vi "Initialize Queue Log.vi"(7 "context":string, 8 "error in (no error)":errorcluster, 9 "queue in (default: new queue)":refnum<queue>, 10 "level":T1 items=["OFF"=0, "FATAL"=100, "ERROR"=200, "WARN"=300, "INFO"=400, "DEBUG"=500, "TRACE"=600, "ALL"=65535]) -> (0 "error out":errorcluster, 1 "queue out":refnum<queue>, 3 "Queue Log Provider out":refnum<class "Queue Log Provider.lvclass">)   [LabVIEW 2019, in "Queue Log Provider.lvclass"]
uses:
  Queue Log Provider.lvclass
  Log Service/public/level.ctl
  Log Service/Log Service.lvclass
  impl/log_message.ctl
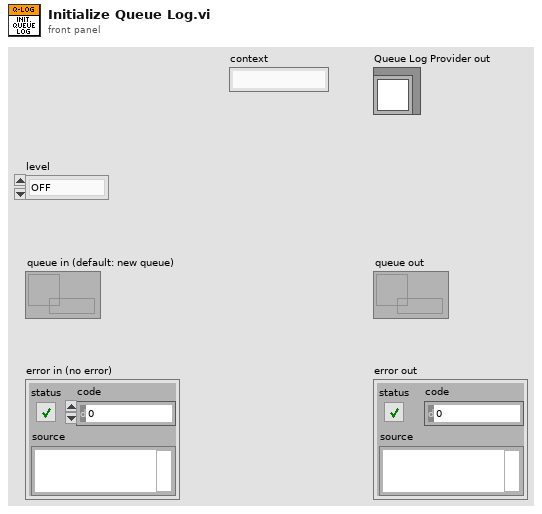
[diagram p1: front panel]
types:
  T1 = typedef "Utility API.lvlib/Log Service.lvclass/level.ctl" = u16
  T2 = typedef "Queue Log Provider.lvclass/log_message.ctl" = cluster{"Time Stamp":timestamp, "level":T1, "context":string, "message":string}
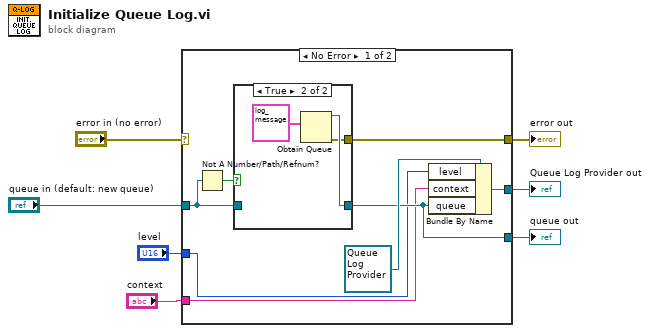
[diagram p0: block diagram]
diagram:
  n1 = case shown="No Error" "error in (no error)" {
    selector: "error in (no error)" -> [_ w21]
    tunnel: [w14 _] -> w7
    tunnel: [w13 w21] -> w6
    tunnel: [w12 w20] -> w5
    tunnel: "queue in (default: new queue)" -> [w11 w20]
    tunnel: "level" -> [w10 _]
    tunnel: "context" -> [w9 _]
    frame No Error {
      n2 = Not A Number/Path/Refnum?(number/path/refnum=w11) -> (NaN/Path/Refnum?=w8:bool)
      n3 = case shown="True" w8 {
        tunnel: [w16 w18] -> w12
        tunnel: w11 -> [w16 _]
        tunnel: [_ w17] -> w13
        frame False {
        }
        frame True {
          n4 = Obtain Queue(element data type=T2 {"Time Stamp"=timestamp(0 s since 1904-01-01), "level"=0, "context"="", "message"=""} ("message")) -> (queue out=w18:refnum<queue>, error out=w17:errorcluster)  [unwired: 4 in, 1 out]
        }
      }
      n5 = Bundle By Name(cluster=refnum<class "Queue Log Provider.lvclass"> refnum ("Queue Log Provider in"), "level"=w10, "context"=w9, "queue"=w12) -> (w14:refnum<class "Queue Log Provider.lvclass">)
    }
    frame Error {
    }
  }
  "Queue Log Provider out" <- w7
  "error out" <- w6
  "queue out" <- w5
